vi "init.vi"(8 "error in (no error)":errorcluster, 11 "PressureTransducerCompensator_Axial in":refnum<class "PressureTransducerCompensator_Axial.lvclass">) -> (0 "error out":errorcluster, 3 "PressureTransducerCompensator_Axial out":refnum<class "PressureTransducerCompensator_Axial.lvclass">)   [LabVIEW 2013, in "PressureTransducerCompensator_Axial.lvclass"]
uses:
  PressureTransducerCompensator_Axial.lvclass
  Configuration/PressureTransducerCompensator.ctl
  Configuration/PIDGains.ctl
  Configuration/PressureTransducerOutputRange.ctl
  PressureTransducerCompensator/PressureTransducerCompensator.lvclass/PressureTransducerCompensator.ctl
  ConfigurationThisComponent/ConfigurationThisComponent.lvclass
  PressureTransducerCompensator/PressureTransducerCompensator.lvclass
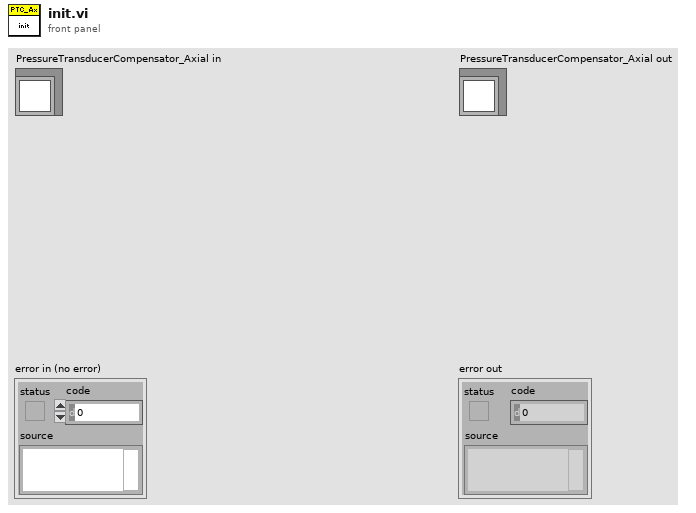
[diagram p1: front panel]
types:
  T1 = typedef "PressureTransducerCompensator.ctl" = cluster{"PID Gains":T2, "Pressure Transducer Output Range":T3, "Vcoil":dbl[unit]}
  T2 = typedef "PIDGains.ctl" = cluster{"Proportional Gain (Kc)":dbl, "Integral Time (Ti, min)":dbl, "Derivative Time (Td, min)":dbl}
  T3 = typedef "PressureTransducerOutputRange.ctl" = cluster{"High":dbl[unit], "Low":dbl[unit]}
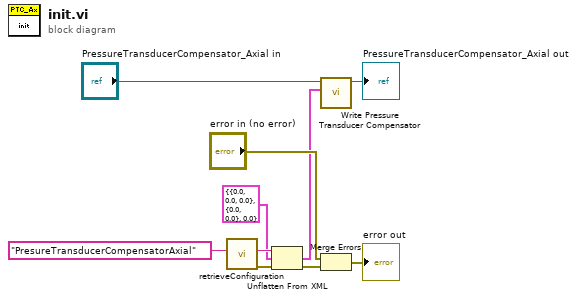
[diagram p0: block diagram]
diagram:
  n1 = call "retrieveConfiguration.vi"("configName"="PresureTransducerCompensatorAxial") -> ("error out"=w8:errorcluster, "xmlConfig"=w7:string)  [unwired: 8 in, 1 out]
  n2 = Unflatten From XML(xml string=w7, type=T1 {"PID Gains"={"Proportional Gain (Kc)"=0.0, "Integral Time (Ti, min)"=0.0, "Derivative Time (Td, min)"=0.0}, "Pressure Transducer Output Range"={"High"=0.0, "Low"=0.0}, "Vcoil"=0.0} ("Pressure Transducer Compensator"), error in (no error)=w8) -> (value=w2:T1, error out=w10:errorcluster)
  n3 = call "Write Pressure Transducer Compensator.vi"("Pressure Transducer Compensator"=w2, "PressureTransducerCompensator in"="PressureTransducerCompensator_Axial in") -> ("PressureTransducerCompensator out"=→"PressureTransducerCompensator_Axial out":refnum<class "PressureTransducerCompensator_Axial.lvclass">)  [unwired: 9 in]
  n4 = Merge Errors("error in (no error)", w10) -> (→"error out":errorcluster)
